vi "Test Effeciency of Position.vi"(9 "Test Voltages":string[](array[string]), 10 "Position":u32, 11 "Efficiency Test in":refnum<class "Efficiency Test.lvclass">) -> (3 "Effeciency Passed":bool)   [LabVIEW 2015, in "Efficiency Test.lvclass"]
uses:
  Efficiency Test.lvclass
  <vilib>/Cree, Inc/Cree Test Framework/Core Launcher/Core Manager Methods -- Enum.ctl
  <vilib>/Cree, Inc/Cree Test Framework/Core Launcher/Core Launcher.lvlib
  <vilib>/Cree, Inc/Cree Test Framework/Classes/Variable Engine/Class/Variable Engine.lvclass
  Test Class/Test Class.lvclass
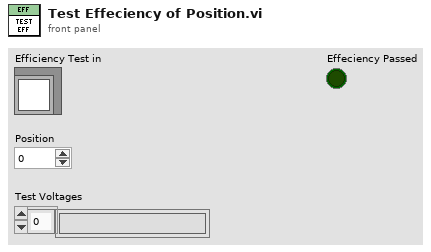
[diagram p1: front panel]
types:
  T1 = typedef "Core Launcher.lvlib/Core Manager Methods -- Enum.ctl" = enum16{"Spawn Objects", "Get Objects", "Destroy Objects"}
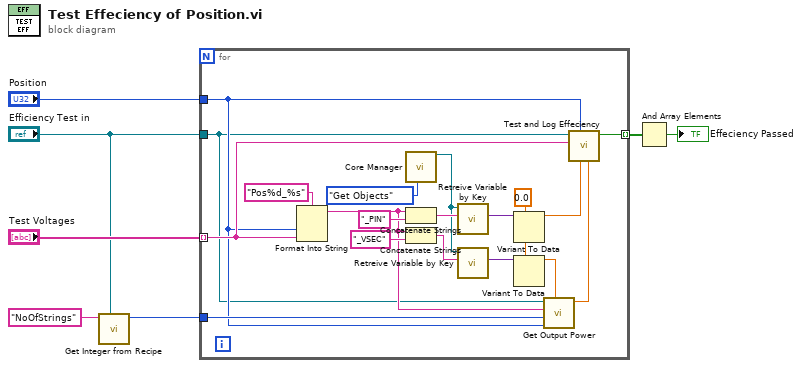
[diagram p0: block diagram]
diagram:
  n1 = call "Get Integer from Recipe.vi"("Test Class in"="Efficiency Test in", "Name"="NoOfStrings" ("Message ('')")) -> ("Value"=w6:i32)  [unwired: 7 in, 2 out]
  n2 = for {
    tunnel: "Test Voltages" -> [w13] mode=indexing
    tunnel: w6 -> [w11]
    tunnel: "Position" -> [w9]
    tunnel: "Efficiency Test in" -> [w8]
    tunnel: [w15] -> w3 mode=indexing
    w18 = 0.0
    n3 = Format Into String(format string="Pos%d_%s", w9, w13) -> (resulting string=w10:string)  [unwired: 2 in, 1 out]
    n4 = call <vilib>:"Core Manager.vi"("Method"=Core_Manager_Methods_--_Enum."Get Objects") -> ("Variable Engine"=w20:refnum<class "Variable Engine.lvclass">)  [unwired: 6 in, 4 out]
    n5 = Concatenate Strings(w10, "_PIN" ("string")) -> (w21:string)
    n6 = Concatenate Strings(w10, "_VSEC" ("string")) -> (w24:string)
    n7 = call <vilib>:"Retreive Variable by Key.vi"("Key"=w21, "Acrobat Template in"=w20) -> ("Value"=w19:variant)  [unwired: 7 in, 2 out]
    n8 = call <vilib>:"Retreive Variable by Key.vi"("Key"=w24, "Acrobat Template in"=w20) -> ("Value"=w23:variant)  [unwired: 7 in, 2 out]
    n9 = Variant To Data(type=w18, Variant=w19) -> (data=w17:dbl)  [unwired: 1 in, 1 out]
    n10 = Variant To Data(type=w18, Variant=w23) -> (data=w12:dbl)  [unwired: 1 in, 1 out]
    n11 = call "Get Output Power.vi"("VSEC"=w12, "Position"=w9, "Number of Strings"=w11, "Test Voltage"=w10, "Efficiency Test"=w8) -> ("Power Out"=w16:dbl)  [unwired: 6 in]
    n12 = call "Test and Log Effeciency.vi"("Power Out"=w16, "Power In"=w17, "Position"=w9, "Test Voltage"=w13, "Efficiency Test"=w8) -> ("Result"=w15:bool)  [unwired: 6 in]
  }
  n13 = And Array Elements(Boolean array=w3) -> (logical AND=→"Effeciency Passed":bool)
